vi "Obtain Recipient.vi"(8 "error in (no error)":errorcluster, 11 "Caller Endpoint in":refnum<class "Caller Endpoint.lvclass">) -> (0 "error out":errorcluster, 2 "Recipient Enqueuer":refnum<class "Message Enqueuer.lvclass">, 3 "Caller Endpoint out":refnum<class "Caller Endpoint.lvclass">)   [LabVIEW 2020, in "Caller Endpoint.lvlib" / "Caller Endpoint.lvclass"]
doc: "This override launches the nested actor specified for this Caller Endpoint, and returns its enqueuer. The endpoint will forward any message it receives from its remote counterpart to this nested actor."
uses:
  <vilib>/NI/Actors/Network Endpoint Actors/Caller Endpoint/Caller Endpoint/Caller Endpoint.lvclass
  C:/Program Files (x86)/National Instruments/LabVIEW 2020/vi.lib/ActorFramework/Actor/Actor.lvclass
  <vilib>/ActorFramework/Message Enqueuer/Message Enqueuer.lvclass
  <vilib>/NI/Actors/Network Endpoint Actors/Caller Endpoint/Caller Endpoint/Caller Endpoint.lvclass/Caller Endpoint.ctl
  <vilib>/ActorFramework/Actor/Actor.lvclass
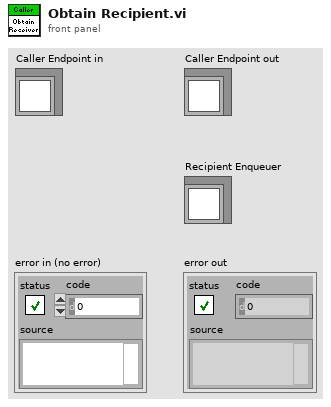
[diagram p1: front panel]
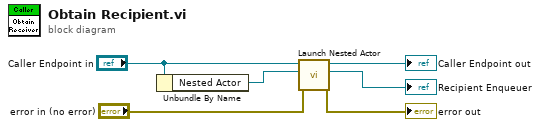
[diagram p0: block diagram]
diagram:
  n1 = Unbundle By Name("Caller Endpoint in") -> ("Nested Actor"=w3:refnum<class "Actor.lvclass">)
  n2 = call <vilib>:"Launch Nested Actor.vi"("error in (no error)"="error in (no error)", "Nested Actor"=w3, "Caller Actor in"="Caller Endpoint in") -> ("error out"=→"error out":errorcluster, "Nested Actor's Enqueuer"=→"Recipient Enqueuer":refnum<class "Message Enqueuer.lvclass">, "Caller Actor out"=→"Caller Endpoint out":refnum<class "Caller Endpoint.lvclass">)  [unwired: 6 in]
